vi "admin tables.vi"() -> ()   [LabVIEW 2020]
uses:
  Data.PG.lvclass
panel:
  in  "End":timestamp
  in  "Start":timestamp
  in  "max points":i32
  in  "Get Data":bool
  out "table selected":string
  in  "max characters (if string)":i32
  in  "new column units":string
  in  "new column name":string
  in  "Create Column":bool
  in  "Ring":u16(ring) items=["double", "string", "integer", "timestamp"]
  in  "columns_list":i32(listbox)
  in  "new table name":string
  in  "Create Table":bool
  in  "tables_list":i32(listbox)
  in  "OK":bool
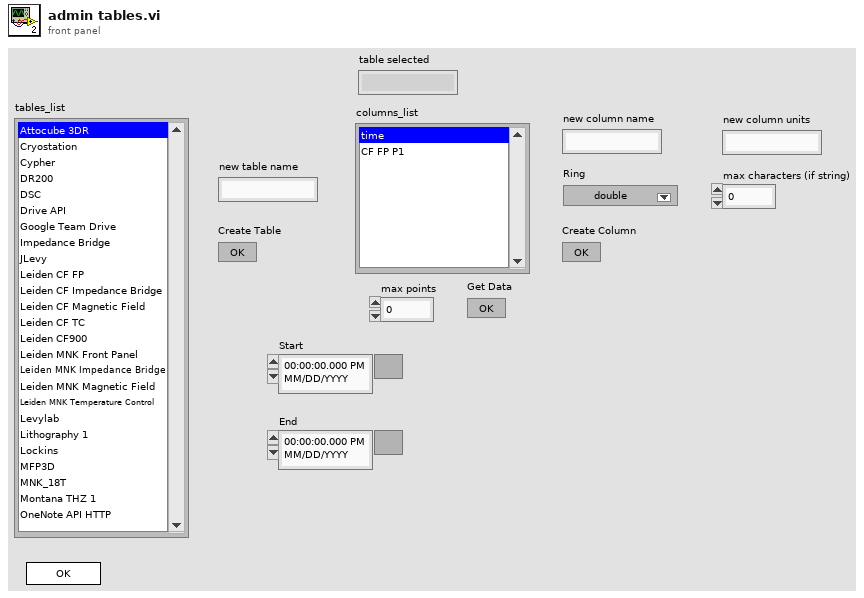
[diagram p1: front panel]
types:
  T1 = enum32{"Invalid", "Standard", "Closed", "Hidden", "Minimized", "Maximized"}
  T2 = enum32{"invalid app kind", "Development System", "Run Time System", "Student Edition", "Embedded LabVIEW", "Evaluation", "Custom"}
  T3 = cluster{"Core":cluster{"Current VI Reference":refnum<vi>, "Close Panel on Exit?":bool}, "Data.PG in":refnum<class "Data.PG.lvclass">, "connection info":cluster{"host":string, "port":string, "dbname":string, "user":string, "password":string}, "table names":string[], "table paths":string[], "column names":string[], "column units":string[], "column paths":string[], "new table name":string, "new column name":string, "new column data type":string, "new column units":string, "selected table":string, "selected column":string, "selected table path":string, "selected column path":string, "Start":timestamp, "End":timestamp, "max points":i32, "selected column units":string}
  T4 = cluster{"host":string, "port":string, "dbname":string, "user":string, "password":string}
  T5 = cluster{"Current VI Reference":refnum<vi>, "Close Panel on Exit?":bool}
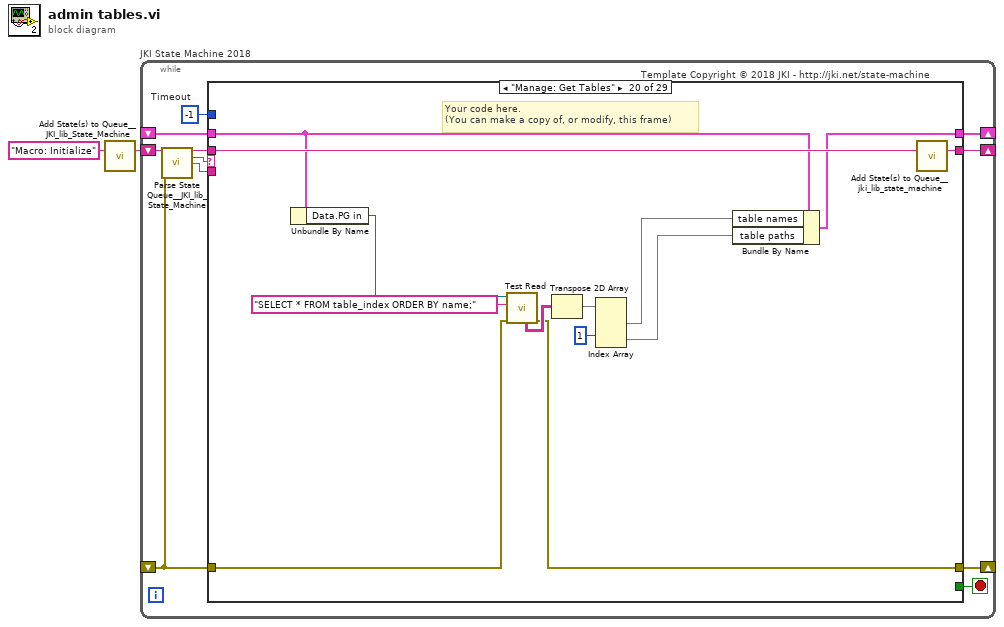
[diagram p0: block diagram]
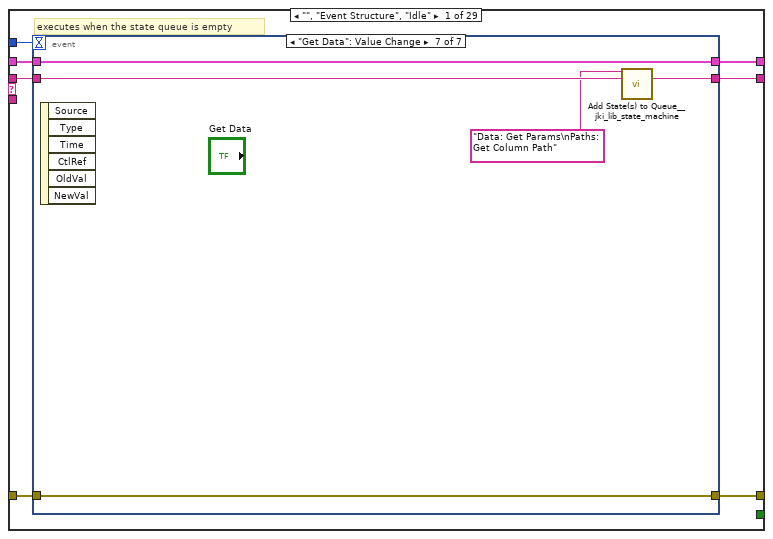
[diagram p2: hidden frame]
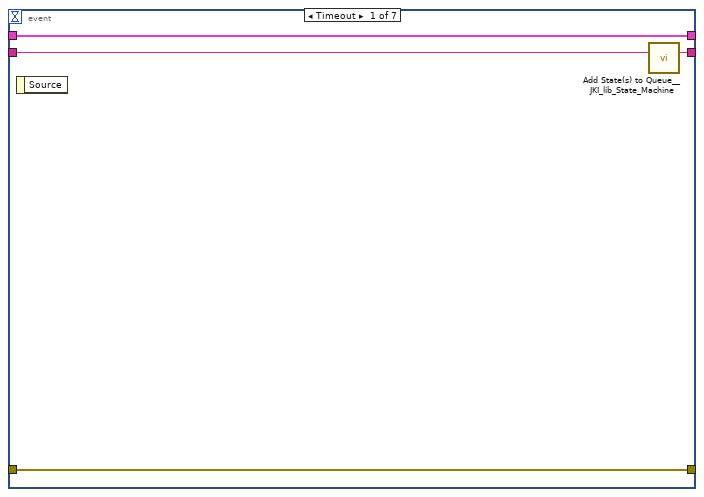
[diagram p3: hidden frame]
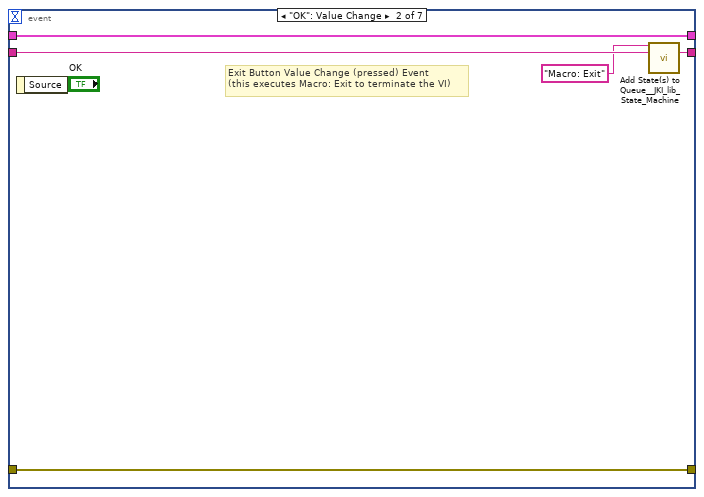
[diagram p4: hidden frame]
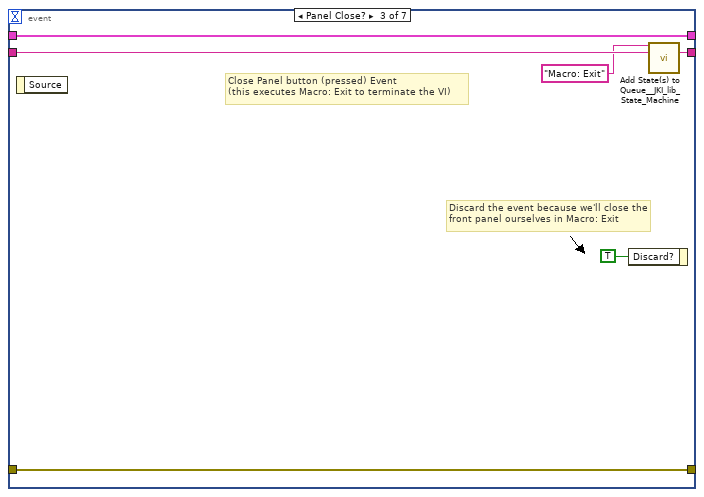
[diagram p5: hidden frame]
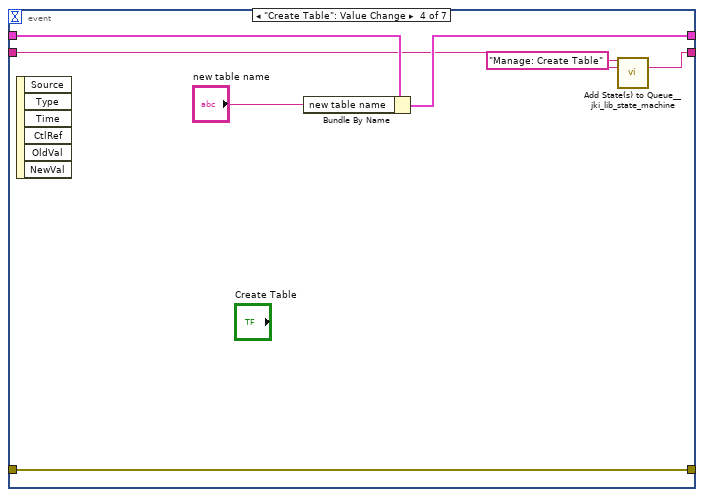
[diagram p6: hidden frame]
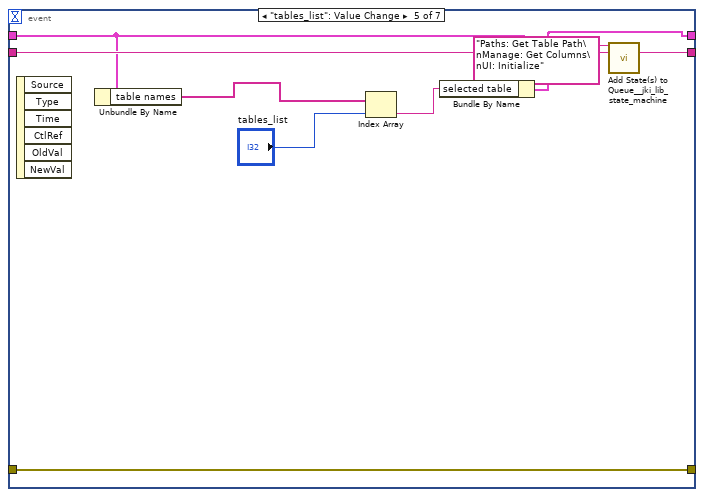
[diagram p7: hidden frame]
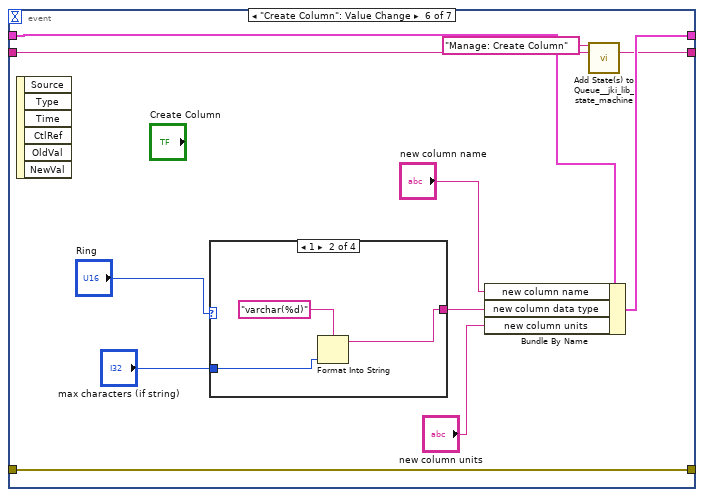
[diagram p8: hidden frame]
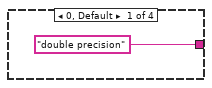
[diagram p9: hidden frame]
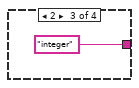
[diagram p10: hidden frame]
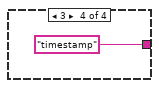
[diagram p11: hidden frame]
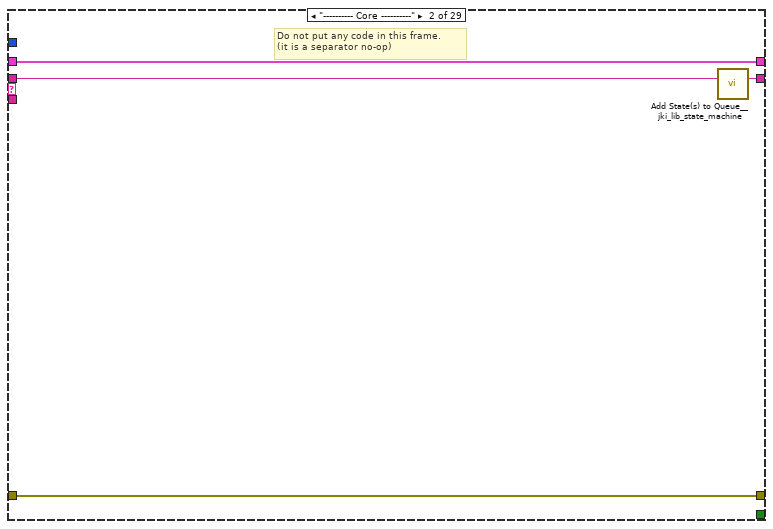
[diagram p12: hidden frame]
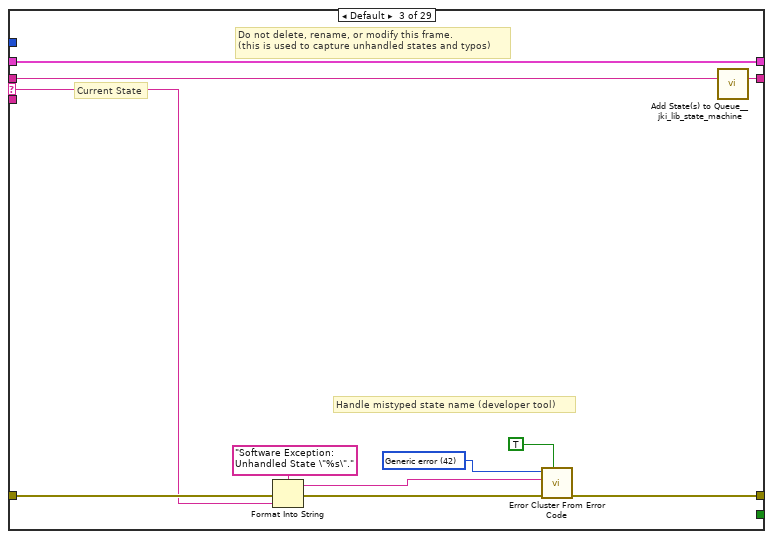
[diagram p13: hidden frame]
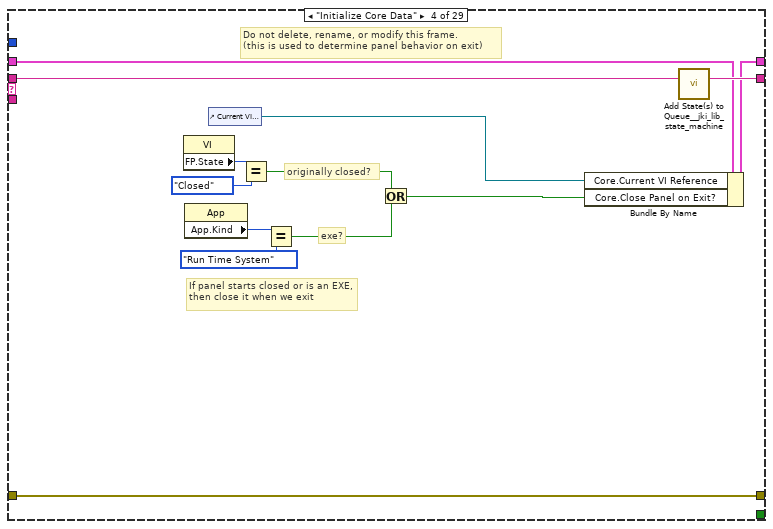
[diagram p14: hidden frame]
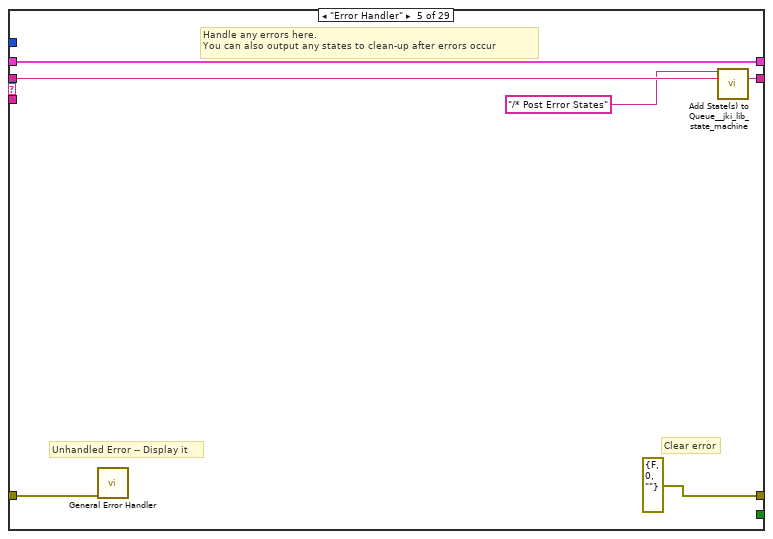
[diagram p15: hidden frame]
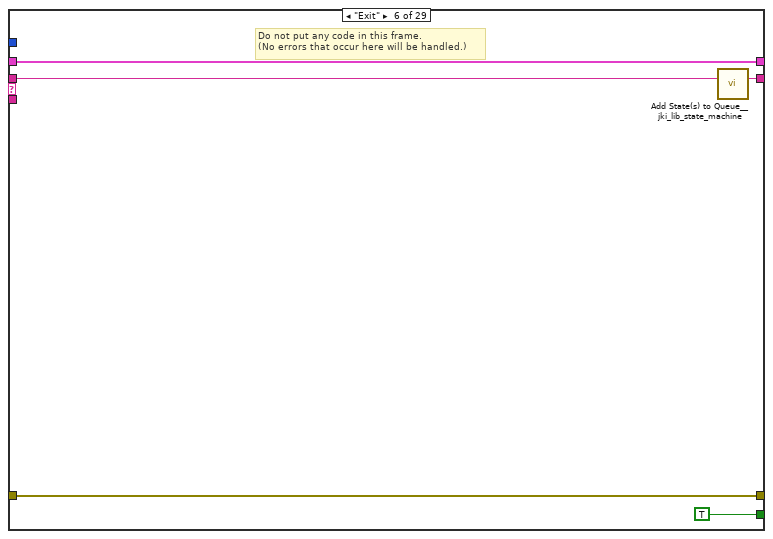
[diagram p16: hidden frame]
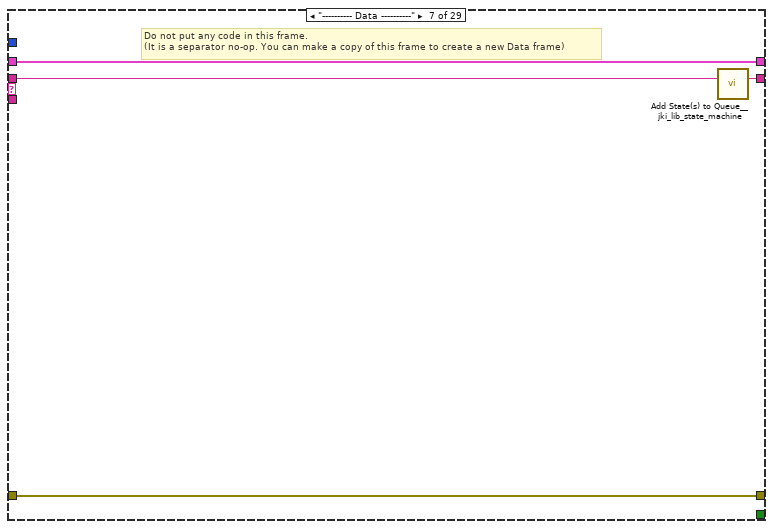
[diagram p17: hidden frame]
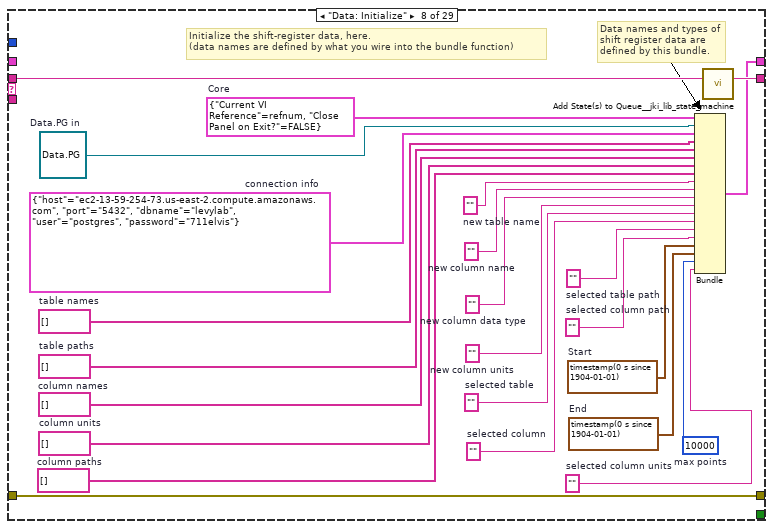
[diagram p18: hidden frame]
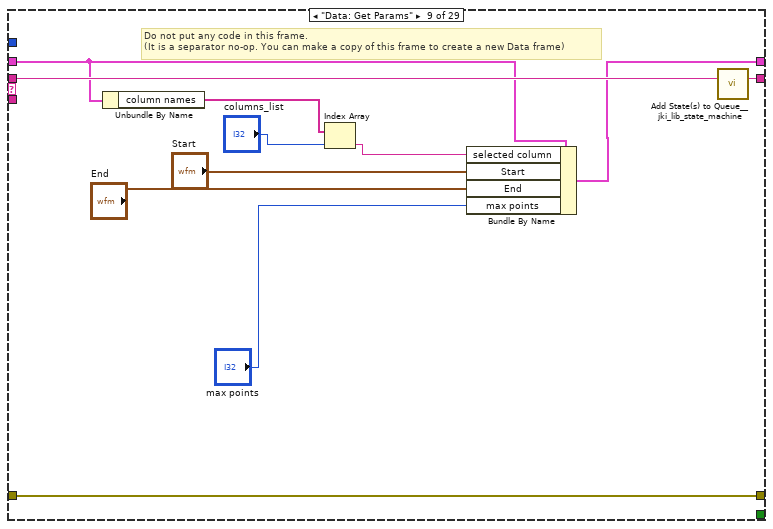
[diagram p19: hidden frame]
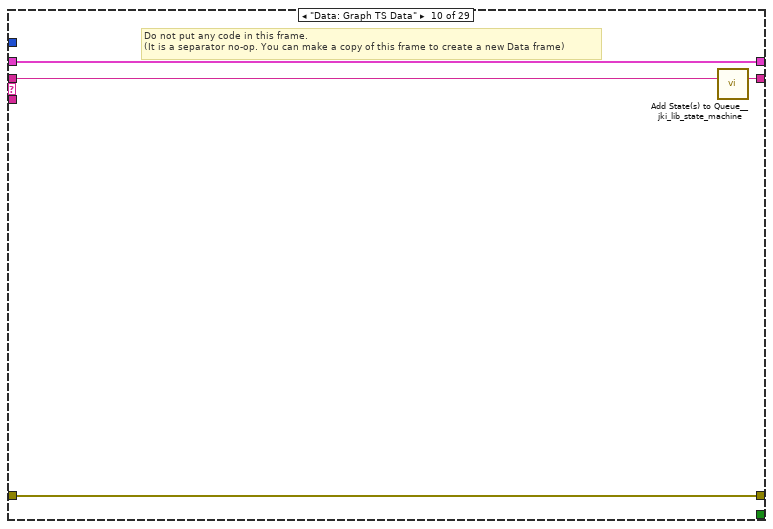
[diagram p20: hidden frame]
diagram:
  n1 = call <vilib>:"Add State(s) to Queue__JKI_lib_State_Machine.vi"("State(s) in (\"\")"="Macro: Initialize") -> ("States Out"=w2:string)  [unwired: 14 in]
  n2 = while "JKI State Machine 2018" {
    shift-right: [w6] -> _
    shift-left: _ -> [w5]
    shift-right: [w9] -> _
    shift-left: _ -> [w3]
    shift-right: [w8] -> _
    shift-left: w2 -> [w10]
    stop <- w7 stop-if-true
    w4 = -1  # Timeout
    # "Template Copyright © 2018 JKI - http://jki.net/state-machine"
    n3 = call <vilib>:"Parse State Queue__JKI_lib_State_Machine.vi"("State Queue"=w10, "Error In (no error)"=w3) -> ("Remaining States"=w12:string, "Current State"=w13:string, "Arguments"=w11:string)  [unwired: 11 in]
    n4 = case shown="\"Manage: Get Tables\"" w13 {
      selector: w13 -> [_ _ w78 _ _ _ _ _ _ _ _ _ _ _ _ _ _ _ _ _ _ _ _ _ _ _ _ _ _]
      tunnel: w12 -> [w20 w77 w82 w101 w107 w112 w116 w140 w151 w155 w163 w167 w174 w180 w191 w260 w265 w275 w279 w292 w311 w325 w359 w383 w389 w398 w402 w415 w432]
      tunnel: w11 -> [_ _ _ _ _ _ _ _ _ _ _ _ _ w175 w185 _ _ _ _ _ _ _ _ _ _ _ _ _ _]
      tunnel: w5 -> [w18 w74 w80 w94 w104 w110 w113 _ w147 w152 w157 w164 w169 w178 w187 w257 w262 w272 w276 w284 w300 w323 w357 w380 w387 w392 w399 w407 w424]
      tunnel: [w17 w75 w84 w98 errorcluster {"status"=FALSE, "code"=0, "source"=""} ("error out") w109 w114 w137 w149 w153 w158 w165 w172 w176 w188 w258 w263 w273 w277 w286 w294 w312 w343 w381 w384 w393 w400 w403 w420] -> w9
      tunnel: w3 -> [w16 w75 w83 w98 w103 w109 w114 w137 w149 w153 w160 w165 w172 w177 w189 w258 w263 w273 w277 w287 w295 w313 w345 w381 w385 w394 w400 w404 w421]
      tunnel: [w19 w76 w81 w100 w106 w111 w115 w139 w150 w154 w162 w166 w173 w179 w190 w259 w264 w274 w278 w291 w310 w324 w358 w382 w388 w397 w401 w414 w431] -> w8
      tunnel: [_ _ _ _ _ TRUE _ _ _ _ _ _ _ _ _ _ _ _ _ _ _ _ _ _ _ _ _ _ _] -> w7
      tunnel: [w15 w74 w80 w99 w104 w110 w113 w138 w148 w152 w157 w164 w169 w178 w187 w257 w262 w272 w276 w283 w299 w323 w357 w380 w387 w391 w399 w406 w423] -> w6
      tunnel: w4 -> [w14 _ _ _ _ _ _ _ _ _ _ _ _ _ _ _ _ _ _ _ _ _ _ _ _ _ _ _ _]
      frame "", "Event Structure", "Idle" {
        # "executes when the state queue is empty"
        n5 = event shown="[6] \"Get Data\": Value Change" {
          selector: _ -> [_ _ _ _ _ _ _]
          dyn-events: _ -> [_ _ _ _ _ _ _]
          timeout: w14 -> [_ _ _ _ _ _ _]
          tunnel: w20 -> [w24 w29 w35 w38 w49 w53 w70]
          tunnel: [w23 w28 w34 w37 w50 w54 w71] -> w19
          tunnel: w18 -> [w21 w26 w32 w41 w45 w60 w73]
          tunnel: [w22 w27 w33 w42 w51 w55 w72] -> w17
          tunnel: w16 -> [w22 w27 w33 w42 w51 w55 w72]
          tunnel: [w21 w26 w32 w40 w44 w59 w73] -> w15
          event Timeout {
            n6 = event-data() -> ()  [unwired: 1 in, 1 out]
            n7 = call <vilib>:"Add State(s) to Queue__JKI_lib_State_Machine.vi"("State(s) in (\"\")"=w24) -> ("States Out"=w23:string)  [unwired: 14 in]
          }
          event "OK": Value Change {
            # "Exit Button Value Change (pressed) Event\n(this executes Macro: Exit to terminate the VI)"
            n8 = event-data() -> ()  [unwired: 1 in, 1 out]
            n9 = call <vilib>:"Add State(s) to Queue__JKI_lib_State_Machine.vi"("State(s) in Front (\"\")"="Macro: Exit", "State(s) in (\"\")"=w29) -> ("States Out"=w28:string)  [unwired: 13 in]
          }
          event Panel Close? {
            # "Discard the event because we'll close the front panel ourselves in Macro: Exit"
            # "Close Panel button (pressed) Event\n(this executes Macro: Exit to terminate the VI)"
            n10 = event-data() -> ()  [unwired: 1 in, 1 out]
            n11 = event-data("Discard?"=TRUE) -> ()  [unwired: 1 in, 1 out]
            n12 = call <vilib>:"Add State(s) to Queue__JKI_lib_State_Machine.vi"("State(s) in Front (\"\")"="Macro: Exit", "State(s) in (\"\")"=w35) -> ("States Out"=w34:string)  [unwired: 13 in]
          }
          event "Create Table": Value Change {
            n13 = event-data() -> ()  [unwired: 1 in, 6 out]
            n14 = Bundle By Name(cluster=w41, "new table name"="new table name") -> (w40:T3)
            n15 = call <vilib>:"Add State(s) to Queue__jki_lib_state_machine.vi"("State(s) in Front (\"\")"="Manage: Create Table" ("State(s) in Front (\"\")"), "State(s) in (\"\")"=w38) -> ("States Out"=w37:string)  [unwired: 13 in]
          }
          event "tables_list": Value Change {
            n16 = event-data() -> ()  [unwired: 1 in, 6 out]
            n17 = Unbundle By Name(w45) -> ("table names"=w46:string[])
            n18 = Index Array(array=w46, index="tables_list") -> (element=w43:string)
            n19 = Bundle By Name(cluster=w45, "selected table"=w43) -> (w44:T3)
            n20 = call <vilib>:"Add State(s) to Queue__jki_lib_state_machine.vi"("State(s) in Front (\"\")"="Paths: Get Table Path\nManage: Get Columns\nUI: Initialize" ("State(s) in Front (\"\")"), "State(s) in (\"\")"=w49) -> ("States Out"=w50:string)  [unwired: 13 in]
          }
          event "Create Column": Value Change {
            n21 = event-data() -> ()  [unwired: 1 in, 6 out]
            n22 = case shown="1" "Ring" {
              tunnel: ["double precision" w64 "integer" "timestamp"] -> w58
              tunnel: "max characters (if string)" -> [_ w65 _ _]
              frame 0, Default {
              }
              frame 1 {
                n23 = Format Into String(format string="varchar(%d)", w65) -> (resulting string=w64:string)  [unwired: 2 in, 1 out]
              }
              frame 2 {
              }
              frame 3 {
              }
            }
            n24 = Bundle By Name(cluster=w60, "new column name"="new column name", "new column data type"=w58, "new column units"="new column units") -> (w59:T3)
            n25 = call <vilib>:"Add State(s) to Queue__jki_lib_state_machine.vi"("State(s) in Front (\"\")"="Manage: Create Column" ("State(s) in Front (\"\")"), "State(s) in (\"\")"=w53) -> ("States Out"=w54:string)  [unwired: 13 in]
          }
          event "Get Data": Value Change {
            n26 = event-data() -> ()  [unwired: 1 in, 6 out]
            n27 = call <vilib>:"Add State(s) to Queue__jki_lib_state_machine.vi"("State(s) in Front (\"\")"="Data: Get Params\nPaths: Get Column Path" ("State(s) in Front (\"\")"), "State(s) in (\"\")"=w70) -> ("States Out"=w71:string)  [unwired: 13 in]
          }
        }
      }
      frame "---------- Core ----------" {
        # "Do not put any code in this frame.\n(it is a separator no-op)"
        n28 = call <vilib>:"Add State(s) to Queue__jki_lib_state_machine.vi"("State(s) in (\"\")"=w77) -> ("States Out"=w76:string)  [unwired: 14 in]
      }
      frame Default {
        w87 = 42 items=["No error", "Argument error", "Memory is full", "Out of zone", "End of file", "File already open", "Generic file I/O error", "File not found", "File permission error", "Disk is full", "Duplicate path", "Too many files open", "System feature not enabled", "Resource file not found", "Cannot add resource", "Resource not found", "Image not found", "Image memory error", "Pen does not exist", "Config type invalid", "Config token not found", "Config parse error", "Config memory error", "Bad external code format", "Bad external code offset", "External code not present", "Null window", "Destroy window error", "Null menu", "Print aborted", "Bad print record", "Print driver error", "Windows error during printing", "Memory error during printing", "Print dialog error", "Generic print error", "Invalid device refnum", "Device not found", "Device parameter error", "Device unit error", "Cannot open device", "Device call aborted", "Generic error", "Cancelled by user", "Object ID too low", "Object ID too high", "Object not in heap", "Unknown heap", "Unknown object (invalid DefProc)", "Unknown object (DefProc not in table)", "Message out of range", "Invalid (null) method", "Unknown message", "Manager call not supported", "Bad address", "Network operation in progress", "Network operation timed out", "Connection is busy", "Network attribute not supported", "Network error", "Address in use", "System out of memory", "Connection aborted", "Connection refused", "Not connected", "Already connected", "Connection closed", "Initialization error (interapplication manager)", "Bad occurrence", "Wait on unbound occurrence handler", "Occurrence queue overflow", "Datalog type conflict", "Unused", "Unrecognized type (interapplication manager)", "Memory corrupt", "Failed to make temporary DLL", "Old CIN version", "Drag socket not found", "Failed to load drop-object", "Failed to register OLE object", "Failed to release OLE object", "Format specifier type mismatch", "Unknown format specifier", "Too few format specifiers", "Too many format specifiers", "Scan failed", "Newer CIN version", "Error converting to variant", "Runtime menu error", "Password tampered", "Variant attribute not found", "Incompatible variant data type", "Event data is not available", "Event Store is not present", "Occurrence is not found", "Event Queue is not created", "Event info is not available", "Refnum passed is NULL", "Error retrieving Class GUID", "Error retrieving CoClass GUID", "Error retrieving TypeLib GUID.", "Bad built application magic bytes.", "Specific driver is different from the specific driver associated with the Logical Name.", "There is no session opened to the class driver.", "Max Error", "MAX - Error with config objects", "MAX - Error loading configuration", "MAX - Group not supported"]
        # "Current State"
        # "Do not delete, rename, or modify this frame.\n(this is used to capture unhandled states and typos)"
        # "Handle mistyped state name (developer tool)"
        n29 = Format Into String(format string="Software Exception: Unhandled State \"%s\"." ("message"), error in=w83, w78) -> (resulting string=w86:string, error out=w85:errorcluster)  [unwired: 1 in]
        n30 = call <vilib>:"Error Cluster From Error Code.vi"("show call chain? (False)"=TRUE, "error in (no error)"=w85, "error message (\"\")"=w86, "error code (0)"=w87) -> ("error out"=w84:errorcluster)  [unwired: 5 in]
        n31 = call <vilib>:"Add State(s) to Queue__jki_lib_state_machine.vi"("State(s) in (\"\")"=w82) -> ("States Out"=w81:string)  [unwired: 14 in]
      }
      frame "Initialize Core Data" {
        # "Do not delete, rename, or modify this frame.\n(this is used to determine panel behavior on exit)"
        # "originally closed?"
        # "exe?"
        # "If panel starts closed or is an EXE, then close it when we exit"
        n32 = property class="VI"() -> ("FP.State"=w91:T1)  [unwired: 2 in, 2 out]
        n33 = property class="App"() -> ("App.Kind"=w97:T2)  [unwired: 2 in, 2 out]
        n34 = control-ref of="Current VI Reference"() -> (w92:refnum<vi>)
        n35 = Equal?(x=w91, y=T1."Closed" ("Front Panel Window:State")) -> (x = y?=w89:bool)
        n36 = Equal?(x=w97, y=T2."Run Time System" ("Application:Kind")) -> (x = y?=w95:bool)
        n37 = Or(x=w89, y=w95) -> (x .or. y?=w93:bool)
        n38 = Bundle By Name(cluster=w94, "Core.Current VI Reference"=w92, "Core.Close Panel on Exit?"=w93) -> (w99:T3)
        n39 = call <vilib>:"Add State(s) to Queue__jki_lib_state_machine.vi"("State(s) in (\"\")"=w101) -> ("States Out"=w100:string)  [unwired: 14 in]
      }
      frame "Error Handler" {
        # "Unhandled Error -- Display it"
        # "Handle any errors here.\nYou can also output any states to clean-up after errors occur"
        # "Clear error"
        n40 = call <vilib>:"General Error Handler.vi"("error in (no error)"=w103) -> ()  [unwired: 10 in, 5 out]
        n41 = call <vilib>:"Add State(s) to Queue__jki_lib_state_machine.vi"("State(s) in Front (\"\")"="/* Post Error States", "State(s) in (\"\")"=w107) -> ("States Out"=w106:string)  [unwired: 13 in]
      }
      frame "Exit" {
        # "Do not put any code in this frame.\n(No errors that occur here will be handled.)"
        n42 = call <vilib>:"Add State(s) to Queue__jki_lib_state_machine.vi"("State(s) in (\"\")"=w112) -> ("States Out"=w111:string)  [unwired: 14 in]
      }
      frame "---------- Data ----------" {
        # "Do not put any code in this frame.\n(It is a separator no-op. You can make a copy of this frame to create a new Data frame)"
        n43 = call <vilib>:"Add State(s) to Queue__jki_lib_state_machine.vi"("State(s) in (\"\")"=w116) -> ("States Out"=w115:string)  [unwired: 14 in]
      }
      frame "Data: Initialize" {
        w117 = ""  # selected column units
        w118 = 10000  # max points
        w119 = timestamp(0 s since 1904-01-01)  # End
        w120 = timestamp(0 s since 1904-01-01)  # Start
        w121 = ""  # selected column path
        w122 = ""  # selected table path
        w123 = ""  # selected column
        w124 = ""  # selected table
        w125 = ""  # new column units
        w126 = ""  # new column data type
        w127 = ""  # new column name
        w128 = ""  # new table name
        w129 = string[] []  # column paths
        w130 = string[] []  # column units
        w131 = string[] []  # column names
        w132 = string[] []  # table paths
        w133 = string[] []  # table names
        w134 = T4 {"host"="ec2-13-59-254-73.us-east-2.compute.amazonaws.com", "port"="5432", "dbname"="levylab", "user"="postgres", "password"="711elvis"}  # connection info
        w135 = refnum<class "Data.PG.lvclass"> refnum  # Data.PG in
        w136 = T5 {"Current VI Reference"=refnum, "Close Panel on Exit?"=FALSE}  # Core
        # "Data names and types of shift register data are defined by this bundle."
        # "Initialize the shift-register data, here.\n(data names are defined by what you wire into the bundle function)"
        n44 = Bundle("Core"=w136, "Data.PG in"=w135, "connection info"=w134, "table names"=w133, "table paths"=w132, "column names"=w131, "column units"=w130, "column paths"=w129, "new table name"=w128, "new column name"=w127, "new column data type"=w126, "new column units"=w125, "selected table"=w124, "selected column"=w123, "selected table path"=w122, "selected column path"=w121, "Start"=w120, "End"=w119, "max points"=w118, "selected column units"=w117) -> (w138:T3)  [unwired: 1 in]
        n45 = call <vilib>:"Add State(s) to Queue__jki_lib_state_machine.vi"("State(s) in (\"\")"=w140) -> ("States Out"=w139:string)  [unwired: 14 in]
      }
      frame "Data: Get Params" {
        # "Do not put any code in this frame.\n(It is a separator no-op. You can make a copy of this frame to create a new Data frame)"
        n46 = Unbundle By Name(w147) -> ("column names"=w145:string[])
        n47 = Index Array(array=w145, index="columns_list") -> (element=w144:string)
        n48 = Bundle By Name(cluster=w147, "selected column"=w144, "Start"="Start", "End"="End", "max points"="max points") -> (w148:T3)
        n49 = call <vilib>:"Add State(s) to Queue__jki_lib_state_machine.vi"("State(s) in (\"\")"=w151) -> ("States Out"=w150:string)  [unwired: 14 in]
      }
      frame "Data: Graph TS Data" {
        # "Do not put any code in this frame.\n(It is a separator no-op. You can make a copy of this frame to create a new Data frame)"
        n50 = call <vilib>:"Add State(s) to Queue__jki_lib_state_machine.vi"("State(s) in (\"\")"=w155) -> ("States Out"=w154:string)  [unwired: 14 in]
      }
      frame "Data: Cleanup" {
        # "Cleanup any data and references, here.\n(this is called automatically, by the Macro: Exit)"
        n51 = Unbundle By Name(w157) -> ("Core.Current VI Reference"=w161:refnum<vi>)
        n52 = Unbundle By Name(w157) -> ("Data.PG in"=w156:refnum<class "Data.PG.lvclass">)
        n53 = Close Reference(reference=w161, error in (no error)=w160) -> (error out=w159:errorcluster)
        n54 = call-dynamic "Close.vi"("error in (no error)"=w159, "Data.PG in"=w156) -> ("error out"=w158:errorcluster)  [unwired: 8 in, 1 out]
        n55 = call <vilib>:"Add State(s) to Queue__jki_lib_state_machine.vi"("State(s) in (\"\")"=w163) -> ("States Out"=w162:string)  [unwired: 14 in]
      }
      frame "---------- UI ----------" {
        # "Do not put any code in this frame.\n(It is a separator no-op. You can make a copy of this frame to create a new UI frame)"
        n56 = call <vilib>:"Add State(s) to Queue__jki_lib_state_machine.vi"("State(s) in (\"\")"=w167) -> ("States Out"=w166:string)  [unwired: 14 in]
      }
      frame "UI: Initialize" {
        # "Initialize the User Interface, here.\n(this is called automatically, by the Macro: Init)"
        n57 = Unbundle By Name(w169) -> ("table names"=w171:string[], "column names"=w170:string[], "selected table"=→"table selected":string)
        n58 = property on="tables_list" class="LstBox (strict)"("Item Names"=w171) -> ()  [unwired: 2 in, 2 out]
        n59 = property on="columns_list" class="LstBox (strict)"("Item Names"=w170) -> ()  [unwired: 2 in, 2 out]
        n60 = call <vilib>:"Add State(s) to Queue__jki_lib_state_machine.vi"("State(s) in (\"\")"=w174) -> ("States Out"=w173:string)  [unwired: 14 in]
      }
      frame "UI: Cursor Set" {
        # "Argument"
        # "Set and Unset Cursor Busy.\n(Usage: \"UI: Cursor Set >> Busy|Idle\")"
        n61 = case shown="\"Idle\", Default" w175 {
          tunnel: w177 -> [w182 w184]
          tunnel: [w181 w183] -> w176
          frame "Idle", Default {
            n62 = call <vilib>:"Unset Busy.vi"("error in (no error)"=w182) -> ("error out"=w181:errorcluster)  [unwired: 10 in]
          }
          frame "Busy" {
            n63 = call <vilib>:"Set Busy.vi"("error in (no error)"=w184) -> ("error out"=w183:errorcluster)  [unwired: 9 in, 1 out]
          }
        }
        n64 = call <vilib>:"Add State(s) to Queue__jki_lib_state_machine.vi"("State(s) in (\"\")"=w180) -> ("States Out"=w179:string)  [unwired: 14 in]
      }
      frame "UI: Front Panel State" {
        # "Argument"
        # "Set Front Panel Open or Closed\n(Usage: \"UI: Front Panel State >> Open|Close\")"
        n65 = Unbundle By Name(w187) -> ("Core.Current VI Reference"=w186:refnum<vi>)
        n66 = case shown="\"Minimize\", \"Minimized\"" w185 {
          tunnel: w189 -> [w197 w212 w223 w236 w249]
          tunnel: [w199 w213 w225 w238 w251] -> w188
          tunnel: w186 -> [w198 w210 w224 w237 w250]
          frame "Open", "Standard", Default {
            w192 = T1."Standard" ("State")
            n67 = property class="VI"(reference=w198, error in=w197) -> (reference out=w195:refnum<vi>, error out=w196:errorcluster, "FP.State"=w194:T1)
            n68 = Not Equal?(x=w194, y=w192) -> (x != y?=w193:bool)
            n69 = case shown="True" w193 {
              tunnel: [w203 w205] -> w199
              tunnel: w196 -> [w202 w205]
              tunnel: w195 -> [w201 _]
              tunnel: w192 -> [w200 _]
              frame True {
                n70 = invoke class="VI" method="FP.Open"(reference=w201, error in=w202, "Activate"=TRUE, "State"=w200) -> (error out=w203:errorcluster)  [unwired: 1 in, 4 out]
              }
              frame False {
              }
            }
          }
          frame "Close", "Closed" {
            n71 = property class="VI"(reference=w210, error in=w212) -> (reference out=w209:refnum<vi>, error out=w211:errorcluster, "FP.State"=w207:T1)
            n72 = Not Equal?(x=w207, y=T1."Closed" ("Front Panel Window:State")) -> (x != y?=w206:bool)
            n73 = case shown="True" w206 {
              tunnel: [w214 w217] -> w213
              tunnel: w211 -> [w214 w216]
              tunnel: w209 -> [_ w215]
              frame False {
              }
              frame True {
                n74 = invoke class="VI" method="FP.Close"(reference=w215, error in=w216) -> (error out=w217:errorcluster)  [unwired: 1 in, 2 out]
              }
            }
          }
          frame "Hidden", "Hide" {
            w218 = T1."Hidden" ("State")
            n75 = property class="VI"(reference=w224, error in=w223) -> (reference out=w221:refnum<vi>, error out=w222:errorcluster, "FP.State"=w220:T1)
            n76 = Not Equal?(x=w220, y=w218) -> (x != y?=w219:bool)
            n77 = case shown="True" w219 {
              tunnel: [w229 w230] -> w225
              tunnel: w222 -> [w228 w230]
              tunnel: w221 -> [w227 _]
              tunnel: w218 -> [w226 _]
              frame True {
                n78 = invoke class="VI" method="FP.Open"(reference=w227, error in=w228, "State"=w226) -> (error out=w229:errorcluster)  [unwired: 2 in, 4 out]
              }
              frame False {
              }
            }
          }
          frame "Minimize", "Minimized" {
            w231 = T1."Minimized" ("State")
            n79 = property class="VI"(reference=w237, error in=w236) -> (reference out=w234:refnum<vi>, error out=w235:errorcluster, "FP.State"=w233:T1)
            n80 = Not Equal?(x=w233, y=w231) -> (x != y?=w232:bool)
            n81 = case shown="True" w232 {
              tunnel: [w242 w243] -> w238
              tunnel: w235 -> [w241 w243]
              tunnel: w234 -> [w240 _]
              tunnel: w231 -> [w239 _]
              frame True {
                n82 = invoke class="VI" method="FP.Open"(reference=w240, error in=w241, "State"=w239) -> (error out=w242:errorcluster)  [unwired: 2 in, 4 out]
              }
              frame False {
              }
            }
          }
          frame "Maximize", "Maximized" {
            w244 = T1."Maximized" ("State")
            n83 = property class="VI"(reference=w250, error in=w249) -> (reference out=w247:refnum<vi>, error out=w248:errorcluster, "FP.State"=w246:T1)
            n84 = Not Equal?(x=w246, y=w244) -> (x != y?=w245:bool)
            n85 = case shown="True" w245 {
              tunnel: [w255 w256] -> w251
              tunnel: w248 -> [w254 w256]
              tunnel: w247 -> [w253 _]
              tunnel: w244 -> [w252 _]
              frame True {
                n86 = invoke class="VI" method="FP.Open"(reference=w253, error in=w254, "State"=w252) -> (error out=w255:errorcluster)  [unwired: 2 in, 4 out]
              }
              frame False {
              }
            }
          }
        }
        n87 = call <vilib>:"Add State(s) to Queue__jki_lib_state_machine.vi"("State(s) in (\"\")"=w191) -> ("States Out"=w190:string)  [unwired: 14 in]
      }
      frame "---------- Macro ----------" {
        # "Do not put any code in this frame.\n(It is a separator no-op. You can make a copy of this frame to create a new Macro frame)"
        n88 = call <vilib>:"Add State(s) to Queue__jki_lib_state_machine.vi"("State(s) in (\"\")"=w260) -> ("States Out"=w259:string)  [unwired: 14 in]
      }
      frame "Macro: Initialize" {
        w261 = "Data: Initialize\nInitialize Core Data\nConnection: Open\nManage: Get Tables\nUI: Initialize\nUI: Front Panel State >> Open"  # Data: Initialize Initialize Core Data Connection: Open Manage: Get Tables UI: Initialize UI: Front Panel State >> Open
        # "Initialization Macro\n(This is called once, when the VI starts)"
        n89 = call <vilib>:"Add State(s) to Queue__jki_lib_state_machine.vi"("State(s) in Front (\"\")"=w261, "State(s) in (\"\")"=w265) -> ("States Out"=w264:string)  [unwired: 13 in]
      }
      frame "Macro: Exit" {
        # "Exit Macro\n(This is called once, when the VI exits)"
        n90 = Unbundle By Name(w272) -> ("Core.Close Panel on Exit?"=w271:bool)
        n91 = Select(t="UI: Front Panel State >> Close", s=w271, f="") -> (s? t:f=w268:string)
        n92 = call <vilib>:"Add State(s) to Queue__jki_lib_state_machine.vi"("State(s) in (\"\")"=w268, "State(s) at Back (\"\")"="Data: Cleanup\nConnection: Close\nExit") -> ("States Out"=w266:string)  [unwired: 13 in]
        n93 = call <vilib>:"Add State(s) to Queue__jki_lib_state_machine.vi"("State(s) in Front (\"\")"=w266, "State(s) in (\"\")"=w275) -> ("States Out"=w274:string)  [unwired: 13 in]
      }
      frame "---------- Manage ----------" {
        # "Template Separator\n(You can make a copy of, or modify, this frame)"
        n94 = call <vilib>:"Add State(s) to Queue__jki_lib_state_machine.vi"("State(s) in (\"\")"=w279) -> ("States Out"=w278:string)  [unwired: 14 in]
      }
      frame "Manage: Get Tables" {
        # "Your code here.\n(You can make a copy of, or modify, this frame)"
        n95 = Unbundle By Name(w284) -> ("Data.PG in"=w290:refnum<class "Data.PG.lvclass">)
        n96 = call-dynamic "Test Read.vi"("error in (no error)"=w287, "command"="SELECT * FROM table_index ORDER BY name;", "Data.PG in"=w290) -> ("error out"=w286:errorcluster, "Result"=w288:string[][])  [unwired: 3 in, 4 out]
        n97 = Transpose 2D Array(2D array=w288) -> (transposed array=w285:string[][])
        n98 = Index Array(array=w285, index (row) #2=1 ("index (row)")) -> (element #1=w282:string[], element #2=w280:string[])  [unwired: 3 in]
        n99 = Bundle By Name(cluster=w284, "table names"=w282, "table paths"=w280) -> (w283:T3)
        n100 = call <vilib>:"Add State(s) to Queue__jki_lib_state_machine.vi"("State(s) in (\"\")"=w292) -> ("States Out"=w291:string)  [unwired: 14 in]
      }
      frame "Manage: Get Columns" {
        # "Your code here.\n(You can make a copy of, or modify, this frame)"
        n101 = Unbundle By Name(w300) -> ("Data.PG in"=w309:refnum<class "Data.PG.lvclass">, "selected table path"=w307:string)
        n102 = Format Into String(format string="SELECT * FROM %s_index; ", w307) -> (resulting string=w306:string)  [unwired: 2 in, 1 out]
        n103 = call-dynamic "Test Read.vi"("error in (no error)"=w295, "command"=w306, "Data.PG in"=w309) -> ("error out"=w294:errorcluster, "Result"=w305:string[][])  [unwired: 3 in, 4 out]
        n104 = Transpose 2D Array(2D array=w305) -> (transposed array=w304:string[][])
        n105 = Index Array(array=w304, index (row) #1=0 ("index (row)"), index (row) #2=1 ("index (row)"), index (row) #3=2 ("index (row)")) -> (element #1=w298:string[], element #2=w297:string[], element #3=w296:string[])  [unwired: 3 in]
        n106 = Bundle By Name(cluster=w300, "column names"=w298, "column units"=w297, "column paths"=w296) -> (w299:T3)
        n107 = call <vilib>:"Add State(s) to Queue__jki_lib_state_machine.vi"("State(s) in Front (\"\")"="UI: Initialize" ("State(s) in Front (\"\")"), "State(s) in (\"\")"=w311) -> ("States Out"=w310:string)  [unwired: 13 in]
      }
      frame "Manage: Create Table" {
        # "Template Separator\n(You can make a copy of, or modify, this frame)"
        n108 = Unbundle By Name(w323) -> ("table paths"=w315:string[], "Data.PG in"=w322:refnum<class "Data.PG.lvclass">, "new table name"=w319:string)
        n109 = Equal?(x=w315, y=string[] []) -> (x = y?=w316:bool)
        n110 = case shown="False" w316 {
          tunnel: w315 -> [w329 _]
          tunnel: [w326 0] -> w317
          frame False {
            n111 = for {
              tunnel: w329 -> [w333] mode=indexing
              tunnel: [w330] -> w328 mode=indexing
              n112 = String Subset(string=w333, offset (0)=5) -> (substring=w331:string)  [unwired: 1 in]
              n113 = Decimal String To Number(string=w331) -> (number=w330:i32)  [unwired: 2 in, 1 out]
            }
            n114 = Array Max & Min(array=w328) -> (max value=w327:i32)  [unwired: 3 out]
            n115 = Increment(x=w327) -> (x+1=w326:i32)
          }
          frame True {
          }
        }
        n116 = Format Into String(format string="CREATE TABLE llab_%03d(\ntime timestamp);\nCREATE TABLE llab_%03d_index(\nname varchar(100) UNIQUE,\nunits varchar(50),\npath varchar(50) UNIQUE);\nINSERT INTO llab_%03d_index VALUES('time','timestamp','time');\nINSERT INTO table_index VALUES('%s','llab_%03d');\nSELECT create_hypertable('llab_%03d','time');\n", w317, w317, w317, w319, w317, w317) -> (resulting string=w320:string)  [unwired: 2 in, 1 out]
        n117 = call-dynamic "Test Read.vi"("error in (no error)"=w313, "command"=w320, "Data.PG in"=w322) -> ("error out"=w312:errorcluster)  [unwired: 3 in, 5 out]
        n118 = call <vilib>:"Add State(s) to Queue__jki_lib_state_machine.vi"("State(s) in Front (\"\")"="Manage: Get Tables\nUI: Initialize" ("State(s) in Front (\"\")"), "State(s) in (\"\")"=w325) -> ("States Out"=w324:string)  [unwired: 13 in]
      }
      frame "Manage: Create Column" {
        # "Template Separator\n(You can make a copy of, or modify, this frame)"
        n119 = Unbundle By Name(w357) -> ("Data.PG in"=w351:refnum<class "Data.PG.lvclass">, "selected table path"=w339:string, "new column data type"=w340:string, "new column name"=w338:string, "new column units"=w337:string)
        n120 = String Subset(string=w340, length (rest)=1 ("length (rest)")) -> (substring=w353:string)  [unwired: 1 in]
        n121 = Equal?(x=w353, y="\"v\"") -> (x = y?=w354:bool)
        n122 = case shown="True" w354 {
          tunnel: w353 -> [w378 _]
          tunnel: [w378 "s"] -> w336
          frame False {
          }
          frame True {
          }
        }
        n123 = Format Into String(format string="SELECT column_name FROM information_schema.columns WHERE table_name = '%s' AND column_name LIKE '%s%%'", w339, w336) -> (resulting string=w350:string)  [unwired: 2 in, 1 out]
        n124 = call-dynamic "Test Read.vi"("error in (no error)"=w345, "command"=w350, "Data.PG in"=w351) -> ("error out"=w344:errorcluster, "Data.PG out"=w346:refnum<class "Data.PG.lvclass">, "Result"=w349:string[][])  [unwired: 3 in, 3 out]
        n125 = Equal?(x=w349, y=string[][] [] ("Result")) -> (x = y?=w347:bool)
        n126 = case shown="True" w347 {
          tunnel: w349 -> [w362 _]
          tunnel: [w360 0] -> w335
          frame False {
            n127 = Transpose 2D Array(2D array=w362) -> (transposed array=w372:string[][])
            n128 = Index Array(array=w372) -> (element=w365:string[])  [unwired: 2 in]
            n129 = Index Array(array=w365) -> (element=w371:string)  [unwired: 1 in]
            n130 = Equal?(x=w371, y="time") -> (x = y?=w369:bool)
            n131 = Select(t=1.0, s=w369, f=0.0) -> (s? t:f=w368:dbl)
            n132 = Array Subset(array=w365, index=w368) -> (w364:string[])  [unwired: 1 in]
            n133 = for {
              tunnel: w364 -> [w376] mode=indexing
              tunnel: [w373] -> w363 mode=indexing
              n134 = String Subset(string=w376, offset (0)=1) -> (substring=w374:string)  [unwired: 1 in]
              n135 = Decimal String To Number(string=w374) -> (number=w373:i32)  [unwired: 2 in, 1 out]
            }
            n136 = Array Max & Min(array=w363) -> (max value=w361:i32)  [unwired: 3 out]
            n137 = Increment(x=w361) -> (x+1=w360:i32)
          }
          frame True {
          }
        }
        n138 = Format Into String(format string="ALTER TABLE %s ADD COLUMN %s%03d %s;\nINSERT INTO %s_index VALUES('%s','%s','%s%03d');", w339, w336, w335, w340, w339, w338, w337, w336, w335) -> (resulting string=w342:string)  [unwired: 2 in, 1 out]
        n139 = call-dynamic "Test Read.vi"("error in (no error)"=w344, "command"=w342, "Data.PG in"=w346) -> ("error out"=w343:errorcluster)  [unwired: 3 in, 5 out]
        n140 = call <vilib>:"Add State(s) to Queue__jki_lib_state_machine.vi"("State(s) in (\"\")"=w359) -> ("States Out"=w358:string)  [unwired: 14 in]
      }
      frame "---------- Connection ----------" {
        # "Template Separator\n(You can make a copy of, or modify, this frame)"
        n141 = call <vilib>:"Add State(s) to Queue__jki_lib_state_machine.vi"("State(s) in (\"\")"=w383) -> ("States Out"=w382:string)  [unwired: 14 in]
      }
      frame "Connection: Close" {
        # "Template Separator\n(You can make a copy of, or modify, this frame)"
        n142 = Unbundle By Name(w387) -> ("Data.PG in"=w386:refnum<class "Data.PG.lvclass">)
        n143 = call-dynamic "Close.vi"("error in (no error)"=w385, "Data.PG in"=w386) -> ("error out"=w384:errorcluster)  [unwired: 8 in, 1 out]
        n144 = call <vilib>:"Add State(s) to Queue__jki_lib_state_machine.vi"("State(s) in (\"\")"=w389) -> ("States Out"=w388:string)  [unwired: 14 in]
      }
      frame "Connection: Open" {
        # "Template Separator\n(You can make a copy of, or modify, this frame)"
        n145 = Unbundle By Name(w392) -> ("Data.PG in"=w396:refnum<class "Data.PG.lvclass">, "connection info"=w395:T4)
        n146 = call "Set Connection Info.vi"("error in (no error)"=w394, "connection info"=w395, "Data.PG in"=w396) -> ("error out"=w393:errorcluster, "Data.PG out"=w390:refnum<class "Data.PG.lvclass">)  [unwired: 7 in]
        n147 = Bundle By Name(cluster=w392, "Data.PG in"=w390) -> (w391:T3)
        n148 = call <vilib>:"Add State(s) to Queue__jki_lib_state_machine.vi"("State(s) in (\"\")"=w398) -> ("States Out"=w397:string)  [unwired: 14 in]
      }
      frame "---------- Paths ----------" {
        # "Template Separator\n(You can make a copy of, or modify, this frame)"
        n149 = call <vilib>:"Add State(s) to Queue__jki_lib_state_machine.vi"("State(s) in (\"\")"=w402) -> ("States Out"=w401:string)  [unwired: 14 in]
      }
      frame "Paths: Get Table Path" {
        # "Template Separator\n(You can make a copy of, or modify, this frame)"
        n150 = Unbundle By Name(w407) -> ("Data.PG in"=w412:refnum<class "Data.PG.lvclass">, "selected table"=w410:string)
        n151 = Format Into String(format string="SELECT path FROM table_index WHERE name='%s'", w410) -> (resulting string=w411:string)  [unwired: 2 in, 1 out]
        n152 = call-dynamic "Test Read.vi"("error in (no error)"=w404, "command"=w411, "Data.PG in"=w412) -> ("error out"=w403:errorcluster, "Result"=w409:string[][])  [unwired: 3 in, 4 out]
        n153 = Index Array(array=w409) -> (element=w408:string[])  [unwired: 2 in]
        n154 = Index Array(array=w408) -> (element=w405:string)  [unwired: 1 in]
        n155 = Bundle By Name(cluster=w407, "selected table path"=w405) -> (w406:T3)
        n156 = call <vilib>:"Add State(s) to Queue__jki_lib_state_machine.vi"("State(s) in (\"\")"=w415) -> ("States Out"=w414:string)  [unwired: 14 in]
      }
      frame "Paths: Get Column Path" {
        # "Template Separator\n(You can make a copy of, or modify, this frame)"
        n157 = Unbundle By Name(w424) -> ("Data.PG in"=w429:refnum<class "Data.PG.lvclass">, "selected table path"=w427:string, "selected column"=w419:string)
        n158 = Format Into String(format string="SELECT path,units FROM %s_index WHERE name='%s'", w427, w419) -> (resulting string=w428:string)  [unwired: 2 in, 1 out]
        n159 = call-dynamic "Test Read.vi"("error in (no error)"=w421, "command"=w428, "Data.PG in"=w429) -> ("error out"=w420:errorcluster, "Result"=w426:string[][])  [unwired: 3 in, 4 out]
        n160 = Index Array(array=w426) -> (element=w425:string[])  [unwired: 2 in]
        n161 = Index Array(array=w425, index #1=0 ("index"), index #2=1 ("index")) -> (element #1=w422:string, element #2=w416:string)
        n162 = Bundle By Name(cluster=w424, "selected column path"=w422, "selected column units"=w416) -> (w423:T3)
        n163 = call <vilib>:"Add State(s) to Queue__jki_lib_state_machine.vi"("State(s) in (\"\")"=w432) -> ("States Out"=w431:string)  [unwired: 14 in]
      }
    }
  }
